vi "手动.vi"() -> ()   [LabVIEW 2017]
uses:
  <vilib>/Platform/TimedLoop/XDataNode/timing_clust.ctl
  <vilib>/Platform/TimedLoop/XDataNode/nitl_modes.ctl
  <vilib>/Platform/TimedLoop/XDataNode/wakeup.ctl
  <vilib>/myRIO/Instrument Drivers/Onboard IO/PWM/vis/Set Duty Cycle and Frequency.vi
  <vilib>/myRIO/Common/Instrument Driver Framework/myRIO v1.0/UART/vis/myRIO v1.0 Close UART.vi
  <vilib>/Utility/error.llb/Error Cluster From Error Code.vi
  <vilib>/myRIO/Common/Instrument Driver Framework/myRIO v1.0/Encoder/vis/myRIO v1.0 Read Encoder.vi
  <vilib>/myRIO/Common/Instrument Driver Framework/myRIO v1.0/DIO/vis/myRIO v1.0 Write DIO.vi
  <vilib>/myRIO/Common/Instrument Driver Framework/myRIO v1.0/PWM/vis/myRIO v1.0 Write PWM.vi
  <vilib>/rvi/errors/niLvFpgaAdjustHostInterfaceError.vi
  <vilib>/FPGAPlugInAG/Dynamic/niLvFpga_Close_Dynamic.vi
  <vilib>/myRIO/Common/Instrument Driver Framework/Utilities/vis/FPGA Ref Manager.vi
  <vilib>/myRIO/Common/Instrument Driver Framework/myRIO v1.0/myRIO v1.0 Reset FPGA.vi
  <vilib>/myRIO/Common/Instrument Driver Framework/myRIO v1.0/IRQ/vis/myRIO v1.0 IRQ Info FGV.vi
  <vilib>/myRIO/Common/Instrument Driver Framework/myRIO v1.0/IRQ/vis/myRIO v1.0 Timer IRQ Info FGV.vi
  <vilib>/myRIO/Common/Instrument Driver Framework/myRIO v1.0/IRQ/vis/myRIO v1.0 ISR Agent.vi
  <vilib>/Platform/TimedLoop/XDataNode/XDataNode.xnode
  <vilib>/rvi/interface/nirviReadWriteControl/nirviReadWriteControl.xnode
  <vilib>/rvi/interface/nirviCloseFPGA/nirviCloseFPGA.xnode
  <vilib>/myRIO/Instrument Drivers/Onboard IO/PWM/PWM.lvlib
  <vilib>/Platform/TimedLoop/XDataNode/XDNodeRunTimeDep.lvlib
  <vilib>/myRIO/Instrument Drivers/Utilities/Utilities.lvlib
  <vilib>/myRIO/Instrument Drivers/Onboard IO/Encoder/Encoder.lvlib
  <vilib>/myRIO/Instrument Drivers/Onboard IO/DIO/DIO.lvlib
  NiFpgaLv.dll
  <vilib>/rvi/interface/Simulation/niFpgaSimulationCallBeginRW.vi
panel:
  in  "Values":bool[](array[boolean])
  in  "PWM":dbl[](array[numeric])
  in  "B DIO7":bool
  out "timed out?":bool
  out "pulse width (uSec)":dbl format="%.2f"
  out "ENC2":i32
  out "ENC1":i32
  out "数组":i32[](array[numeric])
  out "斯必得":dbl[](array[numeric]) format="%#_6f"
  in  "停止":bool
  # "3"
  # "底盘"
  # "夹具"
  # "上下"
  # "4"
  # "夹手"
  # "上下"
  # "1"
  # "底盘4"
  # "2"
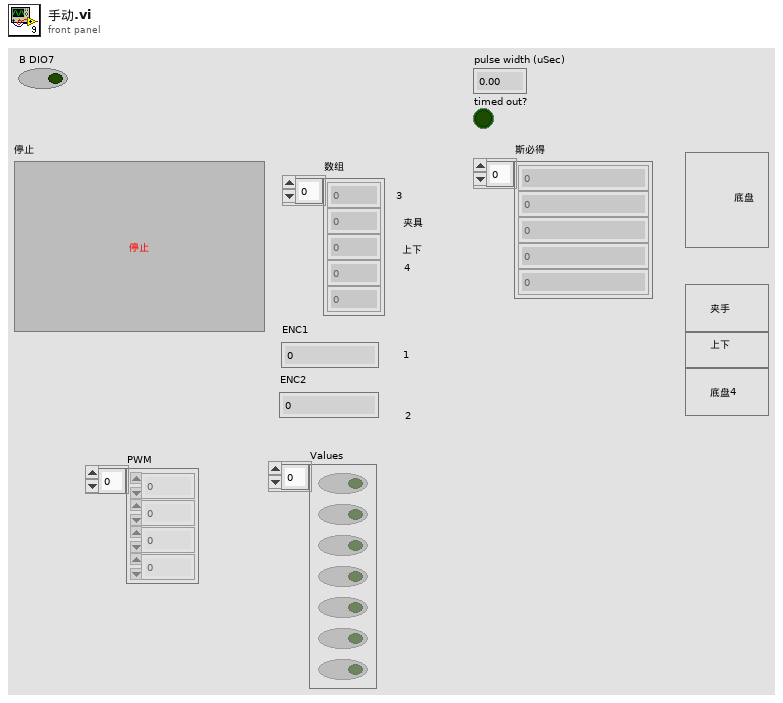
[diagram p1: front panel]
types:
  T1 = typedef "PWM.lvlib/PWM Reference.ctl" = cluster{"myRIO Reference":T2, "PWM Channels Enum":T6, "PWM Configuration":T7}
  T2 = typedef "myRIO Generic Hardware Reference.ctl" = cluster{"myRIO Model":T3, "myRIO Hardware Reference":T4}
  T3 = typedef "Hardware Version Enum.ctl" = enum16{"Unknown", "myRIO-1900", "myRIO-1950", "roboRIO", "NI ELVIS RIO CM"}
  T4 = typedef "myRIO v1.0 Reference.ctl" = cluster{"Generic FPGA Reference":T5, "Allow multiple opens":bool}
  T5 = typedef "Generic FPGA Reference.ctl" = refnum<k20>
  T6 = typedef "PWM Channels Enum.ctl" = enum16{"Not Connected", "C/PWM0", "C/PWM1", "A/PWM0", "A/PWM1", "A/PWM2", "B/PWM0", "B/PWM1", "B/PWM2", "PWM/PWM0", "PWM/PWM1", "PWM/PWM2", "PWM/PWM3", "PWM/PWM4", "PWM/PWM5", "PWM/PWM6", "PWM/PWM7", "PWM/PWM8", "PWM/PWM9"}
  T7 = typedef "PWM.lvlib/PWM Configuration.ctl" = cluster{"Frequency":dbl, "Duty Cycle":dbl}
  T8 = typedef "Encoder.lvlib/Encoder Reference.ctl" = cluster{"myRIO Reference":T2, "Encoder Channels Enum":T9}
  T9 = typedef "Encoder Channels Enum.ctl" = enum16{"Not Connected", "C/ENC0", "C/ENC1", "A/ENC", "B/ENC", "DIO/ENC0", "DIO/ENC1", "DIO/ENC2", "DIO/ENC3", "DIO/ENC4"}
  T10 = typedef "DIO.lvlib/DIO Reference.ctl" = cluster{"myRIO Reference":T2, "DIO Channels List":T11}
  T11 = typedef "DIO Channels List.ctl" = T12[]
  T12 = typedef "DIO Channels Enum.ctl" = enum16{"Not Connected", "C/DIO0", "C/DIO1", "C/DIO2", "C/DIO3", "C/DIO4", "C/DIO5", "C/DIO6", "C/DIO7", "A/DIO0", "A/DIO1", "A/DIO2", "A/DIO3", "A/DIO4", "A/DIO5", "A/DIO6", "A/DIO7", "A/DIO8", "A/DIO9", "A/DIO10", "A/DIO11", "A/DIO12", "A/DIO13", "A/DIO14", "A/DIO15", "B/DIO0", "B/DIO1", "B/DIO2", "B/DIO3", "B/DIO4", "B/DIO5", "B/DIO6", "B/DIO7", "B/DIO8", "B/DIO9", "B/DIO10", "B/DIO11", "B/DIO12", "B/DIO13", "B/DIO14", "B/DIO15", "LED0", "LED1", "LED2", "LED3", "Button0", "DIO/DIO0", "DIO/DIO1", "DIO/DIO2", "DIO/DIO3", "DIO/DIO4", "DIO/DIO5", "DIO/DIO6", "DIO/DIO7", "DIO/DIO8", "DIO/DIO9", "SPI/CS0", "SPI/CS1", "SPI/CS2", "SPI/CS3", "LED RADIO (Green)", "LED RADIO (Red)", "LED COMM (Green)", "LED COMM (Red)", "LED MODE (Green)", "LED MODE (Red)"}
  T13 = cluster{"PWM":T1[], "ENC":T8[], "DIO":T10, "FPGA VI引用输出":refnum<k20>}
  T14 = typedef "XDNodeRunTimeDep.lvlib/timing_clust.ctl" = cluster{"Expected End [f-1]":u64, "Actual End [f-1]":u64, "Finished Late? [f-1]":bool, "Expected End [i-1]":u64, "Actual End [i-1]":u64, "Finished Late? [i-1]":bool, "Expected Start [i]":u64, "Actual Start [i]":u64, "Expected Start [f]":u64, "Actual Start [f]":u64, "Source Name":string, "Structure Name":string, "Period":i64, "Deadline":i64, "Offset":i64, "Start":i64, "Priority":i32, "Timeout":i32, "Mode":T15, "Wakeup Reason":T16, "Error":errorcluster, "Source Type":string, "Secondary Source Type":string, "Global End Time":u64, "Global Start Time":u64, "Frame Duration":u64, "Iteration Duration":u64, "Assigned CPU":i32, "I/O Scan Engine Mode":u32}
  T15 = typedef "XDNodeRunTimeDep.lvlib/nitl_modes.ctl" = enum32{"No Change", "Process missed periods, maintain original phase", "Discard missed periods, maintain original phase", "Process missed periods, ignore original phase", "Discard missed periods, ignore original phase"}
  T16 = typedef "XDNodeRunTimeDep.lvlib/wakeup.ctl" = enum32{"Normal", "Aborted", "Asynchronous wakeup", "Timing source error", "Timed loop error", "Timeout"}
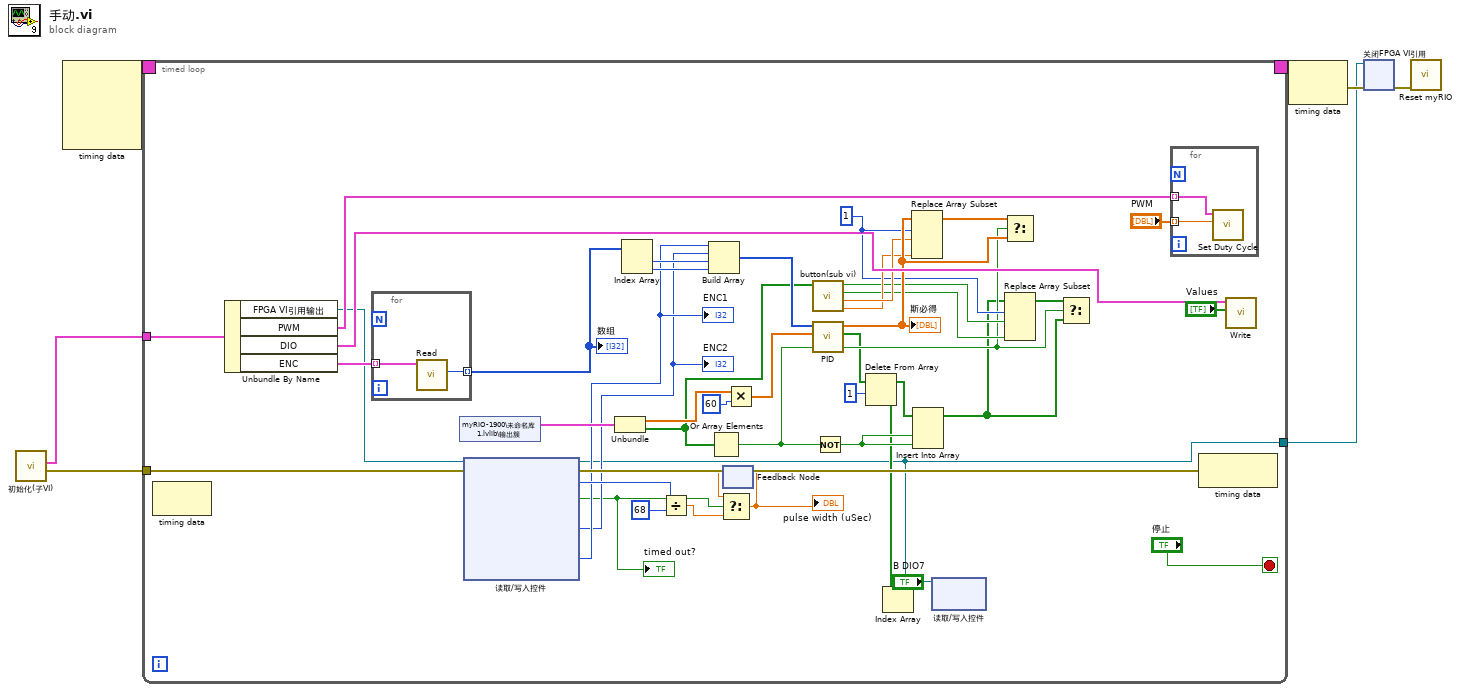
[diagram p0: block diagram]
diagram:
  n1 = call "初始化(子VI).vi"() -> ("ERRO"=w2:errorcluster, "输出簇"=w1:T13)  [unwired: 10 in]
  n2 = node-c288() -> (w7:T14)  [unwired: 4 in]
  n3 = timed-loop {
    timing: w7 -> [_]
    timing-out: [_] -> w6
    tunnel: [w11] -> w3
    tunnel: w2 -> [w26]
    tunnel: w1 -> [w49]
    stop <- "停止" stop-if-true
    w30 = 1 ("索引")
    n4 = node-c288() -> ()  [unwired: 1 in, 1 out]
    n5 = Unbundle By Name(w49) -> ("FPGA VI引用输出"=w24:refnum<k20>, "PWM"=w48:T1[], "DIO"=w46:T10, "ENC"=w47:T8[])
    n6 = for {
      tunnel: [w53] -> w45 mode=indexing
      tunnel: w47 -> [w52] mode=indexing
      n7 = call <vilib>:"Read.vi"("Encoder Ref In"=w52) -> ("Counter Value"=w53:i32)  [unwired: 6 in, 4 out]
    }
    "数组" <- w45
    n8 = shared-variable "myRIO-1900\\未命名库 1.lvlib\\输出簇"() -> (w51:cluster{dbl[], bool[]})  [unwired: 1 in, 1 out]
    n9 = xnode "读取/写入控件"("FPGA VI引用输入"=w24, "错误输入"=w26) -> ("FPGA VI引用输出"=w11:refnum<k20>, "错误输出"=w25:errorcluster, "pulse width (uSec)"=w21:u32, "timed out?"=w16:bool, "ENC 2"=w17:i32, "ENC 1"=w18:i32)  [unwired: 2 in, 1 out]
    "ENC1" <- w18
    "ENC2" <- w17
    "timed out?" <- w16
    n10 = Unbundle(w51) -> (w41:dbl[], w35:bool[])
    n11 = Index Array(array=w45) -> (element #1=w44:i32, element #2=w43:i32)  [unwired: 2 in]
    n12 = Divide(x=w21, y=u32 68) -> (x/y=w19:dbl)
    n13 = Build Array(w18, w17, w44, w43) -> (w42:i32[])
    n14 = Or Array Elements(Boolean array=w35) -> (logical OR=w28:bool)
    n15 = feedback #1() -> (w23:dbl)  [unwired: 1 in]
    n16 = Select(t=w23, s=w16, f=w19) -> (s? t:f=w22:dbl)
    "pulse width (uSec)" <- w22
    n17 = feedback-in #1(w22) -> ()
    n18 = Multiply(x=w41, y=60) -> (x*y=w40:dbl[])
    n19 = call "button(sub vi).vi"("1"=w35) -> (0:"2"=w33:dbl, 1:"1"=w34:dbl, 2:"2"=w31:bool, 3:"1"=w32:bool)  [unwired: 7 in]
    n20 = call "PID.vi"("SET"=w40, "ENC"=w42) -> ("DIR"=w15:bool[], "PWM"=w37:dbl[])  [unwired: 8 in]
    "斯必得" <- w37
    n21 = Not(x=w28) -> (.not. x?=w36:bool)
    n22 = Delete From Array(array=w15, length=1 ("长度")) -> (deleted portion=w12:bool[], array with subset deleted=w14:bool[])  [unwired: 1 in]
    n23 = Index Array(array=w12) -> ()  [unwired: 1 in, 1 out]
    n24 = Replace Array Subset(array=w37, new element #1=w34, index #1=w30, new element #2=w33) -> (w38:dbl[])  [unwired: 1 in]
    n25 = Insert Into Array(array=w14, new element #1=w36, new element #2=w36) -> (w27:bool[])  [unwired: 1 in]
    n26 = xnode "读取/写入控件"("FPGA VI引用输入"=w11, "B DIO7"="B DIO7") -> ()  [unwired: 1 in, 2 out]
    n27 = Select(t=w38, s=w28, f=w37) -> ()  [unwired: 1 out]
    n28 = Replace Array Subset(array=w27, new element #1=w32, index #1=w30, new element #2=w31) -> (w29:bool[])  [unwired: 1 in]
    n29 = Select(t=w29, s=w28, f=w27) -> ()  [unwired: 1 out]
    n30 = for {
      tunnel: w48 -> [w55] mode=indexing
      tunnel: "PWM" -> [w54] mode=indexing
      n31 = call <vilib>:"Set Duty Cycle.vi"("Duty Cycle"=w54, "PWM Ref In"=w55) -> ()  [unwired: 7 in, 2 out]
    }
    n32 = node-c288(w25) -> ()  [unwired: 1 out]
    n33 = call <vilib>:"Write.vi"("Values"="Values", "DIO Ref In"=w46) -> ()  [unwired: 7 in, 2 out]
  }
  n34 = node-c288(w6) -> (w5:errorcluster)
  n35 = xnode "关闭FPGA VI引用"("FPGA VI引用输入"=w3, "错误输入"=w5) -> ("错误输出"=w4:errorcluster)
  n36 = call <vilib>:"Reset myRIO.vi"("error in (no error)"=w4) -> ()  [unwired: 10 in, 1 out]
